vi "Get Payoff Matrix.vi"(8 "error in (no error)":errorcluster, 11 "Read From File (F)":bool) -> (0 "error out":errorcluster, 3 "Payoff Matrix":dbl[][](array[numeric]))   [LabVIEW 2015]
uses:
  <vilib>/Utility/file.llb/Read Delimited Spreadsheet (DBL).vi
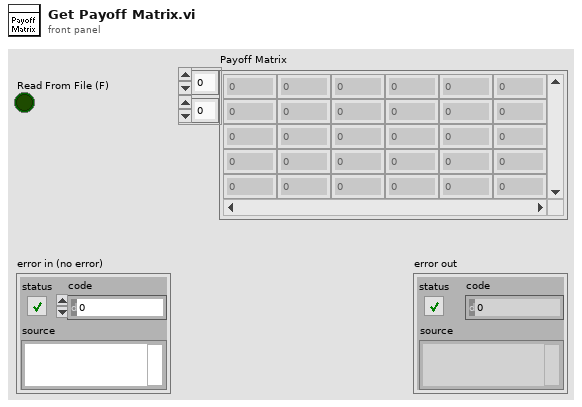
[diagram p1: front panel]
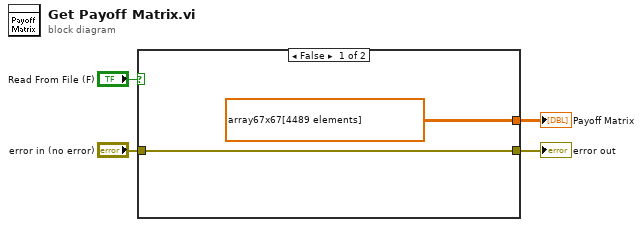
[diagram p0: block diagram]
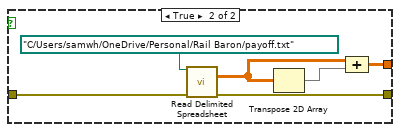
[diagram p2: hidden frame]
diagram:
  n1 = case shown="False" "Read From File (F)" {
    tunnel: "error in (no error)" -> [w5 w11]
    tunnel: [w5 w10] -> w3
    tunnel: [dbl[][] array67x67[4489 elements] ("Payoff Matrix 2") w8] -> w2
    frame False {
    }
    frame True {
      n2 = call-poly <vilib>:"Read Delimited Spreadsheet.vi"("file path (dialog if empty)"=path "C:/Users/samwh/OneDrive/Personal/Rail Baron/payoff.txt", "error in (no error)"=w11) -> ("all rows"=w9:dbl[][], "error out"=w10:errorcluster)  [unwired: 8 in, 4 out]
      n3 = Transpose 2D Array(2D array=w9) -> (transposed array=w7:dbl[][])
      n4 = Compound Arithmetic op=ADD(w9, w7) -> (w8:dbl[][])
    }
  }
  "Payoff Matrix" <- w2
  "error out" <- w3
